vi "mro_open.vi"() -> (0 "error out":errorcluster, 2 "return type":i8, 3 "status":i32)   [LabVIEW 2011]
uses:
  mirao52e.dll
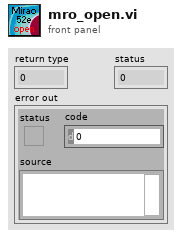
[diagram p1: front panel]
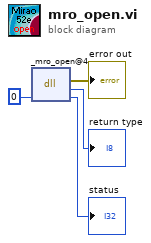
[diagram p0: block diagram]
diagram:
  n1 = dll-call lib="C:/Users/myerslab/Documents/Tests/MiraoWrappers/mirao52e.dll" fn="_mro_open@4"("status"=0) -> (error out=→"error out":errorcluster, "return type"=→"return type":i8, "status"=→"status":i32)  [unwired: 3 in, 1 out]
